vi "Wired Logging Example.vi"() -> ()   [LabVIEW 2018]
uses:
  Log Levels.ctl
  Failure Information.ctl
  Log Record.ctl
  Logger/Internal Log Levels.ctl
  ff44e4a9-c346-414c-ae2a-efcf3ff82913.vi
  Handlers/String Handler/String Handler.lvclass
  C:/Users/Colin/Documents/software_projects/glog/Logging/Handlers/Formatting Handler/Formatting Handler.lvclass
  Logger/Logger.lvclass
  Logging.lvlib
panel:
  out "failure info":T1 {"Log Record"."timestamp" format="%<%x %.3X>T"}
  in  "loop iteration delay [ms]":u32=10
  in  "minimum log level":T4=enum."Info"
  out "error out":errorcluster
  in  "log messages":string
  in  "total iterations":i32=30
  in  "restart logging at":i32=20
  in  "stop logging at":i32=10
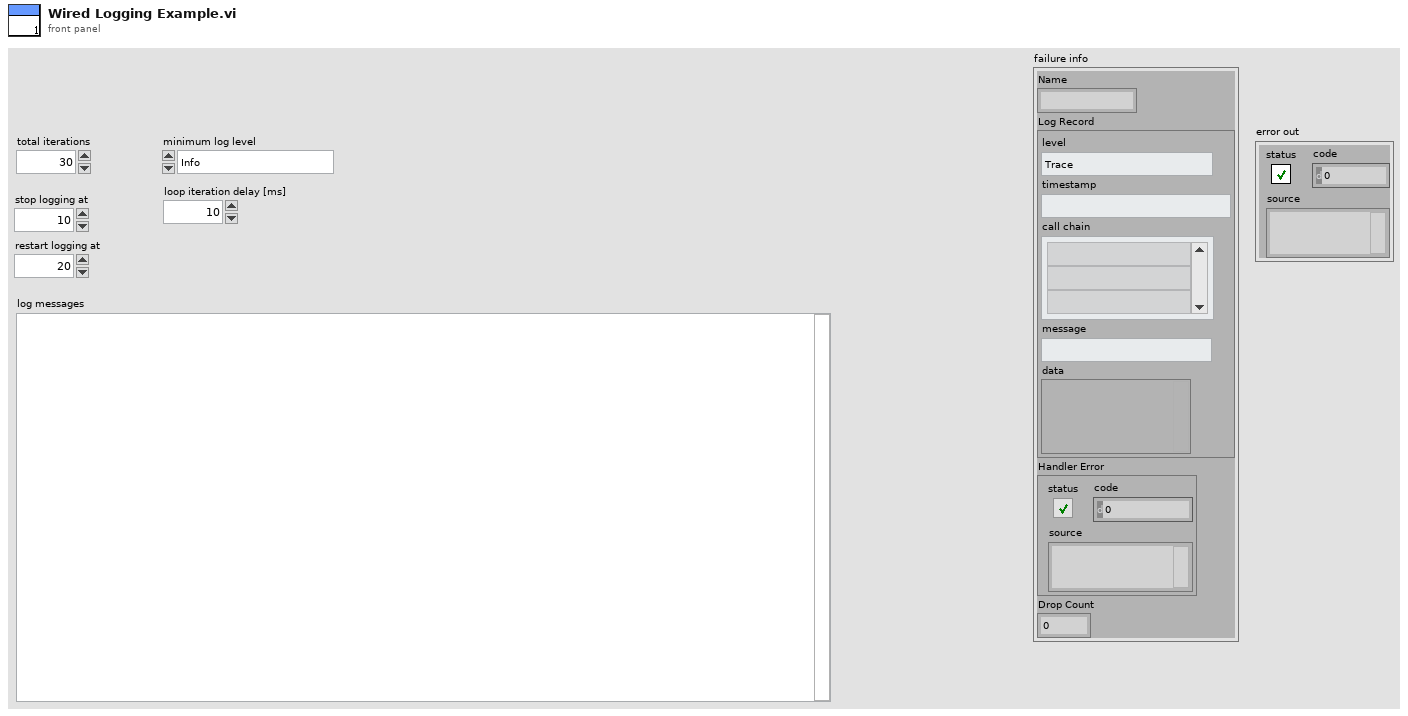
[diagram p1: front panel]
types:
  T1 = typedef "Logging.lvlib/Failure Information.ctl" = cluster{"Name":string, "Log Record":T2, "Handler Error":errorcluster, "Drop Count":u32}
  T2 = typedef "Logging.lvlib/Log Record.ctl" = cluster{"level":T3, "timestamp":timestamp, "call chain":string[], "message":string, "data":variant}
  T3 = typedef "Logging.lvlib/Internal Log Levels.ctl" = enum16{"Trace", "Debug", "Info", "Warning", "Error", "Critical", "Internal"}
  T4 = typedef "Logging.lvlib/Log Levels.ctl" = enum16{"Trace", "Debug", "Info", "Warning", "Error", "Critical"}
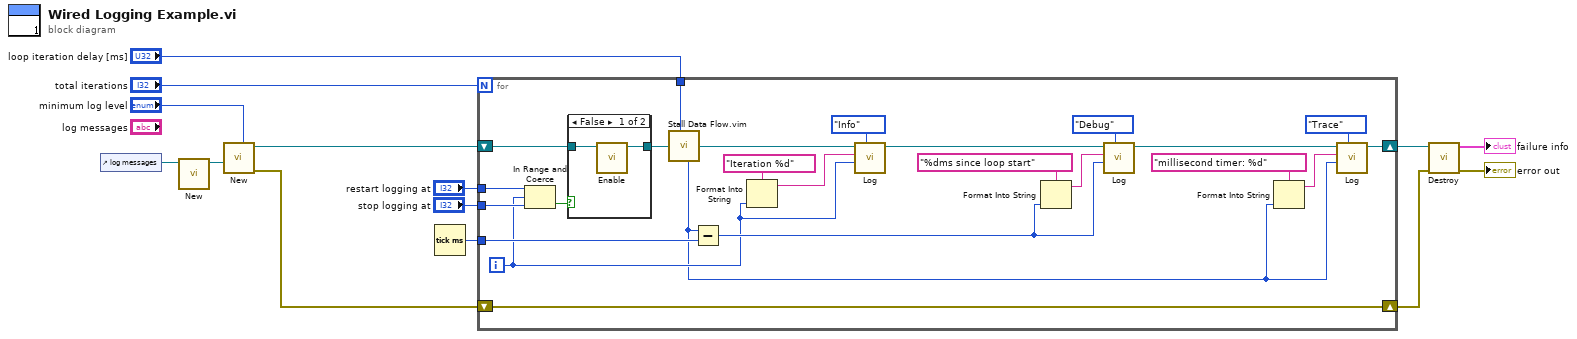
[diagram p0: block diagram]
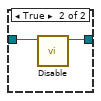
[diagram p2: hidden frame]
diagram:
  n1 = control-ref of="log messages"() -> (w8:refnum<vi>)
  n2 = call "New.vi"("string control"=w8) -> ("new string handler"=w9:refnum<class "String Handler.lvclass">)  [unwired: 10 in]
  n3 = call "New.vi"("minimum log level (Info)"="minimum log level", "log handler (file handler)"=w9) -> ("error out"=w6:errorcluster, "logger"=w14:refnum<class "Logger.lvclass">)  [unwired: 8 in]
  n4 = Tick Count (ms)() -> (millisecond timer value=w13:u32)
  n5 = for {
    N: "total iterations" -> [_]
    shift-right: [w16] -> w7
    shift-left: w14 -> [w30]
    tunnel: w13 -> [w36]
    tunnel: "stop logging at" -> [w32]
    tunnel: "restart logging at" -> [w31]
    shift-right: [w28] -> w5
    shift-left: w6 -> [w28]
    tunnel: "loop iteration delay [ms]" -> [w21]
    i -> [w22]
    n6 = In Range and Coerce(upper limit=w31, x=w22, lower limit=w32) -> (In Range?=w33:bool)  [unwired: 1 out]
    n7 = case shown="False" w33 {
      tunnel: w30 -> [w40 w42]
      tunnel: [w39 w41] -> w29
      frame False {
        n8 = call "Enable.vi"("logger in"=w40) -> ("logger out"=w39:refnum<class "Logger.lvclass">)  [unwired: 10 in]
      }
      frame True {
        n9 = call "Disable.vi"("logger in"=w42) -> ("logger out"=w41:refnum<class "Logger.lvclass">)  [unwired: 10 in]
      }
    }
    n10 = call "Stall Data Flow.vim"("value in"=w29, "milliseconds to wait"=w21) -> ("millisecond timer value"=w15:u32, "value out"=w35:refnum<class "Logger.lvclass">)
    n11 = Subtract(x=w15, y=w36) -> (x-y=w23:u32)
    n12 = Format Into String(format string="Iteration %d" ("message"), w22) -> (resulting string=w26:string)  [unwired: 2 in, 1 out]
    n13 = call "Log.vi"("log level"=Log_Levels."Info", "data (null)"=w22, "message"=w26, "logger in"=w35) -> ("logger out"=w38:refnum<class "Logger.lvclass">)  [unwired: 7 in]
    n14 = Format Into String(format string="%dms since loop start" ("message"), w23) -> (resulting string=w24:string)  [unwired: 2 in, 1 out]
    n15 = call "Log.vi"("log level"=Log_Levels."Debug", "data (null)"=w23, "message"=w24, "logger in"=w38) -> ("logger out"=w17:refnum<class "Logger.lvclass">)  [unwired: 7 in]
    n16 = Format Into String(format string="millisecond timer: %d" ("message"), w15) -> (resulting string=w20:string)  [unwired: 2 in, 1 out]
    n17 = call "Log.vi"("log level"=Log_Levels."Trace", "data (null)"=w15, "message"=w20, "logger in"=w17) -> ("logger out"=w16:refnum<class "Logger.lvclass">)  [unwired: 7 in]
  }
  n18 = call "Destroy.vi"("error in (no error)"=w5, "logger in"=w7) -> ("error out"=→"error out":errorcluster, "failure info"=→"failure info":T1)  [unwired: 8 in]
